vi "Balloon Control.vi"(10 "lines":tag, 11 "Delay (ms)":u32=500) -> ()   [LabVIEW 2020]
uses:
  Controls/Balloon.ctl
  <vilib>/DAQmx/write.llb/DAQmx Write.vi
  <vilib>/DAQmx/write.llb/DAQmx Write (Digital 1D Bool 1Chan 1Samp).vi
  <vilib>/DAQmx/create/channels.llb/DAQmx Create Channel (DO-Digital Output).vi
  <vilib>/DAQmx/miscellaneous.llb/DAQmx Fill In Error Info.vi
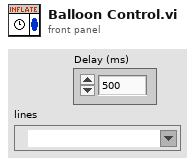
[diagram p1: front panel]
types:
  T1 = typedef "Balloon.ctl" = enum16{"On", "Delay", "Off", "Exit"}
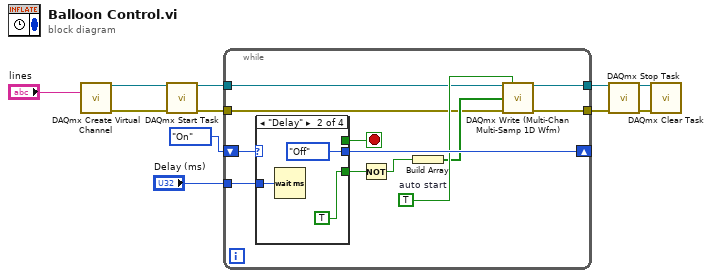
[diagram p0: block diagram]
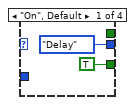
[diagram p2: hidden frame]
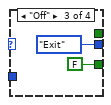
[diagram p3: hidden frame]
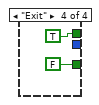
[diagram p4: hidden frame]
diagram:
  n1 = call-poly <vilib>:"DAQmx Create Virtual Channel.vi"("lines"="lines") -> ("task out"=w7:refnum<k21>, "error out"=w8:errorcluster)  [unwired: 13 in]
  n2 = call <vilib>:"DAQmx Start Task.vi"("task/channels in"=w7, "error in"=w8) -> ("task out"=w6:refnum<k21>, "error out"=w5:errorcluster)  [unwired: 12 in]
  n3 = while {
    shift-right: [w22] -> _
    shift-left: Balloon."On" -> [w23]
    tunnel: "Delay (ms)" -> [w20]
    tunnel: [w17] -> w3
    tunnel: [w16] -> w4
    tunnel: w6 -> [w15]
    tunnel: w5 -> [w14]
    stop <- w21 stop-if-true
    w19 = TRUE  # auto start
    n4 = case shown="\"Delay\"" w23 {
      tunnel: [TRUE TRUE FALSE FALSE] -> w13
      tunnel: [Balloon."Delay" Balloon."Off" Balloon."Exit" _] -> w22
      tunnel: [_ _ _ TRUE] -> w21
      tunnel: w20 -> [_ w26 _ _]
      frame "On", Default {
      }
      frame "Delay" {
        n5 = Wait (ms)(milliseconds to wait=w26) -> ()  [unwired: 1 out]
      }
      frame "Off" {
      }
      frame "Exit" {
      }
    }
    n6 = Not(x=w13) -> (.not. x?=w12:bool)
    n7 = Build Array(w12) -> (w18:bool[])
    n8 = call-poly "DAQmx Write (Multi-Chan Multi-Samp 1D Wfm).vi"("task/channels in"=w15, "auto start"=w19, "data"=w18, "error in"=w14) -> ("task out"=w16:refnum<k21>, "error out"=w17:errorcluster)  [unwired: 9 in, 1 out]
  }
  n9 = call <vilib>:"DAQmx Stop Task.vi"("task/channels in"=w4, "error in"=w3) -> ("task out"=w2:refnum<k21>, "error out"=w1:errorcluster)  [unwired: 12 in]
  n10 = call <vilib>:"DAQmx Clear Task.vi"("task in"=w2, "error in"=w1) -> ()  [unwired: 13 in, 1 out]
